vi "单独启动(子VI).vi"(11 "启动模块":T1) -> ()   [LabVIEW 2016, in "质控单元.lvlib"]
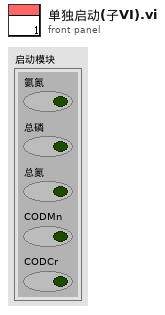
[diagram p1: front panel]
types:
  T1 = cluster{"氨氮":bool, "总磷":bool, "总氮":bool, "CODMn":bool, "CODCr":bool}
  T2 = enum32{"Bad", "Idle", "Run top level", "Running"}
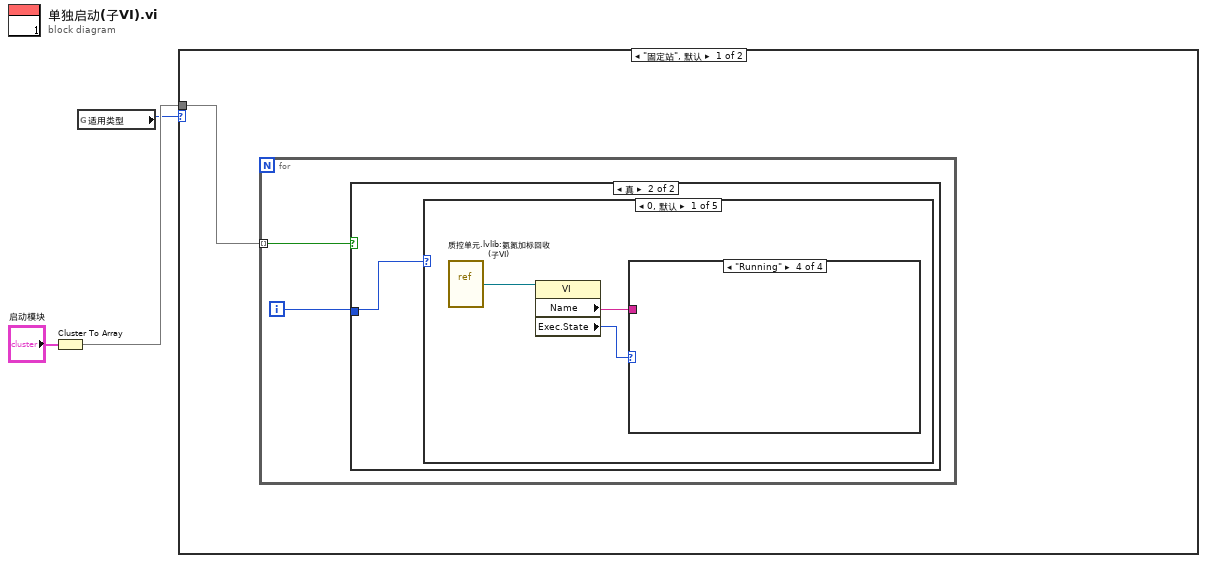
[diagram p0: block diagram]
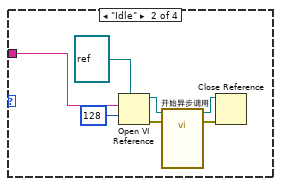
[diagram p4: hidden frame]
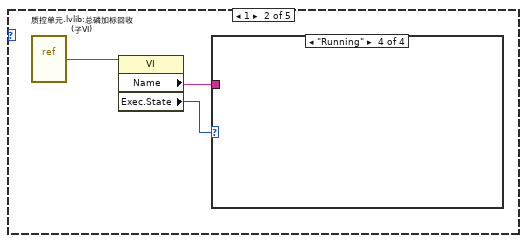
[diagram p6: hidden frame]
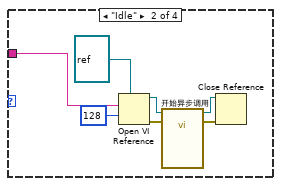
[diagram p8: hidden frame]
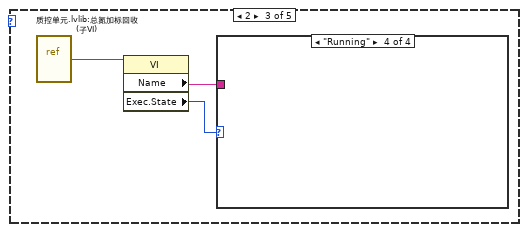
[diagram p10: hidden frame]
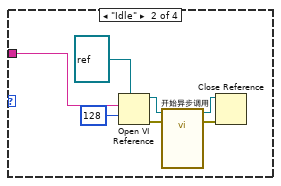
[diagram p12: hidden frame]
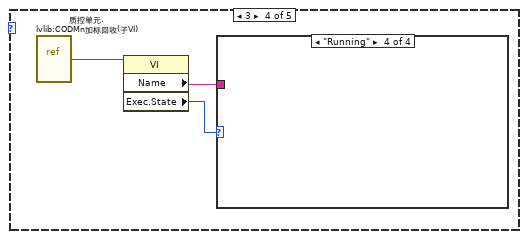
[diagram p14: hidden frame]
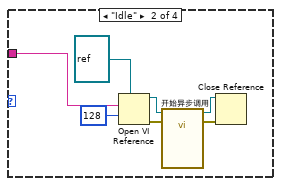
[diagram p16: hidden frame]
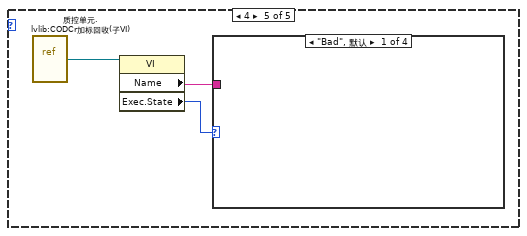
[diagram p18: hidden frame]
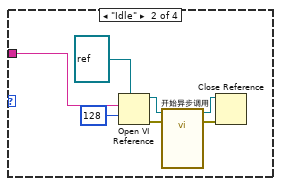
[diagram p19: hidden frame]
diagram:
  n1 = Cluster To Array(cluster="启动模块") -> (array=w2:bool[])
  n2 = global read "断电保存全局.vi" "适用类型"() -> (w1:enum16{"固定站", "微站"})
  n3 = case shown="\"固定站\", 默认" w1 {
    tunnel: w2 -> [w4 w58]
    frame "固定站", Default {
      n4 = for {
        tunnel: w4 -> [w5] mode=indexing
        i -> [w6]
        n5 = case shown="真" w5 {
          tunnel: w6 -> [_ w7]
          frame False {
          }
          frame True {
            n6 = case shown="0, 默认" w7 {
              frame 0, Default {
                n7 = vi-ref "质控单元.lvlib:氨氮加标回收 (子VI).vi"() -> (w10:refnum<vi>)
                n8 = property class="VI"(reference=w10) -> ("Name"=w8:string, "Exec.State"=w9:T2)  [unwired: 1 in, 2 out]
                n9 = case shown="\"Running\"" w9 {
                  tunnel: w8 -> [_ w13 _ _]
                  frame "Bad", Default {
                  }
                  frame "Idle" {
                    n10 = Open VI Reference(type specifier VI Refnum (for type only)=refnum<vi> refnum ("类型说明符VI引用句柄（仅用于类型）"), vi path=w13, options=128 ("选项")) -> (vi reference=w17:refnum<vi>, error out=w12:errorcluster)  [unwired: 3 in]
                    n11 = call-by-ref "开始异步调用"(reference=w17, error in=w12) -> (reference out=w16:refnum<vi>, error out=w11:errorcluster)  [unwired: 12 in]
                    n12 = Close Reference(reference=w16, error in (no error)=w11) -> ()  [unwired: 1 out]
                  }
                  frame "Run top level" {
                  }
                  frame "Running" {
                  }
                }
              }
              frame 1 {
                n13 = vi-ref "质控单元.lvlib:总磷加标回收 (子VI).vi"() -> (w20:refnum<vi>)
                n14 = property class="VI"(reference=w20) -> ("Name"=w18:string, "Exec.State"=w19:T2)  [unwired: 1 in, 2 out]
                n15 = case shown="\"Running\"" w19 {
                  tunnel: w18 -> [_ w23 _ _]
                  frame "Bad", Default {
                  }
                  frame "Idle" {
                    n16 = Open VI Reference(type specifier VI Refnum (for type only)=refnum<vi> refnum ("类型说明符VI引用句柄（仅用于类型）"), vi path=w23, options=128 ("选项")) -> (vi reference=w27:refnum<vi>, error out=w22:errorcluster)  [unwired: 3 in]
                    n17 = call-by-ref "开始异步调用"(reference=w27, error in=w22) -> (reference out=w26:refnum<vi>, error out=w21:errorcluster)  [unwired: 12 in]
                    n18 = Close Reference(reference=w26, error in (no error)=w21) -> ()  [unwired: 1 out]
                  }
                  frame "Run top level" {
                  }
                  frame "Running" {
                  }
                }
              }
              frame 2 {
                n19 = vi-ref "质控单元.lvlib:总氮加标回收 (子VI).vi"() -> (w30:refnum<vi>)
                n20 = property class="VI"(reference=w30) -> ("Name"=w28:string, "Exec.State"=w29:T2)  [unwired: 1 in, 2 out]
                n21 = case shown="\"Running\"" w29 {
                  tunnel: w28 -> [_ w33 _ _]
                  frame "Bad", Default {
                  }
                  frame "Idle" {
                    n22 = Open VI Reference(type specifier VI Refnum (for type only)=refnum<vi> refnum ("类型说明符VI引用句柄（仅用于类型）"), vi path=w33, options=128 ("选项")) -> (vi reference=w37:refnum<vi>, error out=w32:errorcluster)  [unwired: 3 in]
                    n23 = call-by-ref "开始异步调用"(reference=w37, error in=w32) -> (reference out=w36:refnum<vi>, error out=w31:errorcluster)  [unwired: 12 in]
                    n24 = Close Reference(reference=w36, error in (no error)=w31) -> ()  [unwired: 1 out]
                  }
                  frame "Run top level" {
                  }
                  frame "Running" {
                  }
                }
              }
              frame 3 {
                n25 = vi-ref "质控单元.lvlib:CODMn加标回收(子VI).vi"() -> (w40:refnum<vi>)
                n26 = property class="VI"(reference=w40) -> ("Name"=w38:string, "Exec.State"=w39:T2)  [unwired: 1 in, 2 out]
                n27 = case shown="\"Running\"" w39 {
                  tunnel: w38 -> [_ w43 _ _]
                  frame "Bad", Default {
                  }
                  frame "Idle" {
                    n28 = Open VI Reference(type specifier VI Refnum (for type only)=refnum<vi> refnum ("类型说明符VI引用句柄（仅用于类型）"), vi path=w43, options=128 ("选项")) -> (vi reference=w47:refnum<vi>, error out=w42:errorcluster)  [unwired: 3 in]
                    n29 = call-by-ref "开始异步调用"(reference=w47, error in=w42) -> (reference out=w46:refnum<vi>, error out=w41:errorcluster)  [unwired: 12 in]
                    n30 = Close Reference(reference=w46, error in (no error)=w41) -> ()  [unwired: 1 out]
                  }
                  frame "Run top level" {
                  }
                  frame "Running" {
                  }
                }
              }
              frame 4 {
                n31 = vi-ref "质控单元.lvlib:CODCr加标回收(子VI).vi"() -> (w50:refnum<vi>)
                n32 = property class="VI"(reference=w50) -> ("Name"=w48:string, "Exec.State"=w49:T2)  [unwired: 1 in, 2 out]
                n33 = case shown="\"Bad\", 默认" w49 {
                  tunnel: w48 -> [_ w53 _ _]
                  frame "Bad", Default {
                  }
                  frame "Idle" {
                    n34 = Open VI Reference(type specifier VI Refnum (for type only)=refnum<vi> refnum ("类型说明符VI引用句柄（仅用于类型）"), vi path=w53, options=128 ("选项")) -> (vi reference=w57:refnum<vi>, error out=w52:errorcluster)  [unwired: 3 in]
                    n35 = call-by-ref "开始异步调用"(reference=w57, error in=w52) -> (reference out=w56:refnum<vi>, error out=w51:errorcluster)  [unwired: 12 in]
                    n36 = Close Reference(reference=w56, error in (no error)=w51) -> ()  [unwired: 1 out]
                  }
                  frame "Run top level" {
                  }
                  frame "Running" {
                  }
                }
              }
            }
          }
        }
      }
    }
    frame "微站" {
      n37 = global read "断电保存全局.vi" "模块组合"() -> (w59:enum16{"氨氮总磷", "总磷总氮", "氨氮、总磷、总氮"})
      n38 = case shown="\"氨氮、总磷、总氮\"" w59 {
        tunnel: w58 -> [w65 w73 w77]
        frame "氨氮总磷", Default {
          n39 = Index Array(array=w65) -> (element #1=w63:bool, element #2=w62:bool, element #4=w61:bool, element #5=w60:bool)  [unwired: 5 in, 1 out]
          n40 = And(x=w63, y=w62) -> (x .and. y?=w64:bool)
          n41 = case shown="真" w64 {
            tunnel: w63 -> [w67 _]
            tunnel: w62 -> [w66 _]
            frame False {
              # "氨氮或总磷"
              n42 = case shown="真" w67 {
                frame False {
                }
                frame True {
                  n43 = call "氨氮加标回收 (子VI).vi"() -> ()  [unwired: 12 in]
                }
              }
              n44 = case shown="真" w66 {
                frame False {
                }
                frame True {
                  n45 = call "总磷加标回收 (子VI).vi"() -> ()  [unwired: 12 in]
                }
              }
            }
            frame True {
              # "氨氮总磷同时"
              n46 = call "氨氮总磷加标回收 (子VI).vi"() -> ()  [unwired: 12 in]
            }
          }
          n47 = case shown="真" w61 {
            frame False {
            }
            frame True {
              n48 = call "CODMn加标回收(子VI).vi"() -> ()  [unwired: 12 in]
            }
          }
          n49 = case shown="真" w60 {
            frame False {
            }
            frame True {
              n50 = call "CODCr加标回收(子VI).vi"() -> ()  [unwired: 12 in]
            }
          }
        }
        frame "总磷总氮" {
          n51 = Index Array(array=w73) -> (element #1=w68:bool, element #2=w72:bool, element #3=w71:bool, element #4=w70:bool, element #5=w69:bool)  [unwired: 5 in]
          n52 = case shown="真" w70 {
            frame False {
            }
            frame True {
              n53 = call "CODMn加标回收(子VI).vi"() -> ()  [unwired: 12 in]
            }
          }
          n54 = And(x=w72, y=w71) -> (x .and. y?=w74:bool)
          n55 = case shown="真" w74 {
            tunnel: w72 -> [w76 _]
            tunnel: w71 -> [w75 _]
            frame False {
              n56 = case shown="真" w76 {
                frame False {
                }
                frame True {
                  n57 = call "总磷加标回收 (子VI).vi"() -> ()  [unwired: 12 in]
                }
              }
              n58 = case shown="真" w75 {
                frame False {
                }
                frame True {
                  n59 = call "总氮加标回收 (子VI).vi"() -> ()  [unwired: 12 in]
                }
              }
            }
            frame True {
              n60 = call "总磷总氮加标回收 (子VI).vi"() -> ()  [unwired: 12 in]
            }
          }
          n61 = case shown="真" w69 {
            frame False {
            }
            frame True {
              n62 = call "CODCr加标回收(子VI).vi"() -> ()  [unwired: 12 in]
            }
          }
          n63 = case shown="真" w68 {
            frame False {
            }
            frame True {
              n64 = call "氨氮加标回收 (子VI).vi"() -> ()  [unwired: 12 in]
            }
          }
        }
        frame "氨氮、总磷、总氮" {
          n65 = for {
            tunnel: w77 -> [w78] mode=indexing
            i -> [w79]
            n66 = case shown="真" w78 {
              tunnel: w79 -> [_ w80]
              frame False {
              }
              frame True {
                n67 = case shown="1" w80 {
                  frame 0, Default {
                    n68 = call "氨氮加标回收 (子VI).vi"() -> ()  [unwired: 12 in]
                  }
                  frame 1 {
                    n69 = call "总磷加标回收 (子VI).vi"() -> ()  [unwired: 12 in]
                  }
                  frame 2 {
                    n70 = call "总氮加标回收 (子VI).vi"() -> ()  [unwired: 12 in]
                  }
                  frame 3 {
                    n71 = call "CODMn加标回收(子VI).vi"() -> ()  [unwired: 12 in]
                  }
                  frame 4 {
                    n72 = call "CODCr加标回收(子VI).vi"() -> ()  [unwired: 12 in]
                  }
                }
              }
            }
          }
        }
      }
    }
  }
